vi "Get Children.vi"(8 "error in (no error)":errorcluster, 11 "Element Array in":refnum<class "Element Array.lvclass">) -> (0 "error out":errorcluster, 2 "Children":refnum<class "Data Item.lvclass">[](array[class]), 3 "Element Array out":refnum<class "Element Array.lvclass">)   [LabVIEW 2020, in "VILab.lvlib" / "Element Array.lvclass"]
uses:
  Element Array.lvclass
  Data Item/Data Item.lvclass
  Element Array.lvclass/Element Array.ctl
  Attribute/Attribute.lvclass
  C:/Users/User/Documents/LabVIEW Data/Projects/VILab/source/SubVIs/Classes/Data Item/Data Item.lvclass
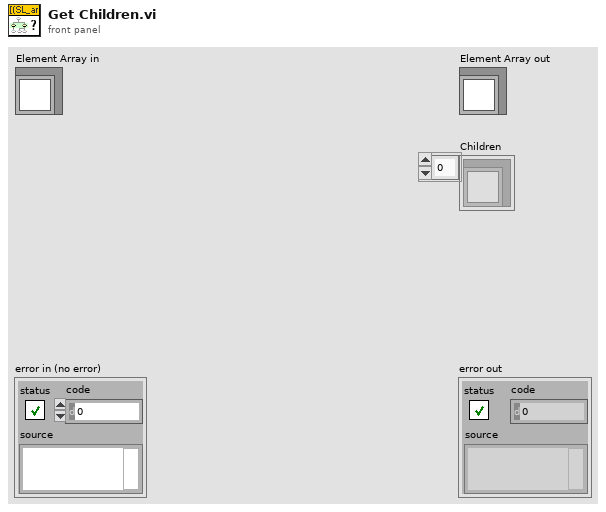
[diagram p1: front panel]
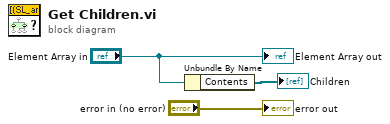
[diagram p0: block diagram]
diagram:
  n1 = Unbundle By Name("Element Array in") -> ("Contents"=→"Children":refnum<class "Attribute.lvclass">[])
  "error out" <- "error in (no error)"
  "Element Array out" <- "Element Array in"
